vi "诊断标定4.vi"(8 "CAN端口":u16(ring), 9 "设备索引号":u16(ring), 10 "CAN卡类型":u32(ring)=4) -> ()   [LabVIEW 2013] (continued)
                n3070 = Build Array(i16 5 ("元素"), w4389, w4383, w4382, w4381, w4380, 0.0 ("元素")) -> (w4393:dbl[])
                n3071 = call "多帧发送机制(EV05).vi"("can卡类型"=w4397, "设备索引号"=w4396, "CAN端口"=w4395, "命令"=w4390, "板号"=u8 0, "命令序号"=w4379, "输入数据"=w4393) -> ()  [unwired: 1 in, 12 out]
              }
            }
            n3072 = local write "命令序号"(w4351) -> ()
            n3073 = local write "命令"(w4356) -> ()
            n3074 = local write "清BUFF"(FALSE ("清BUFF")) -> ()
            n3075 = local write "控制1"(TRUE ("控制1")) -> ()
            n3076 = global write "EV05全局变量1.vi" "流控帧 2"(FALSE ("流控帧 2")) -> ()
            n3077 = local write "写?"(FALSE ("写?")) -> ()
            n3078 = local write "消除"(TRUE ("消除")) -> ()
          }
          frame #2 {
            n3079 = flat-sequence {
              tunnel: [w4399] -> w4398
              tunnel: w4398 -> [w4406]
              frame #0 {
                n3080 = while {
                  tunnel: [w4400] -> w4399
                  i -> [w4404]
                  stop <- w4401 stop-if-true
                  n3081 = local read "继电器超时处理"() -> (w4400:bool)
                  n3082 = Greater Or Equal?(x=w4404, y=20) -> (x >= y?=w4402:bool)
                  n3083 = Wait Until Next ms Multiple(millisecond multiple=u32 100 ("毫秒倍数")) -> ()  [unwired: 1 out]
                  n3084 = Or(x=w4400, y=w4402) -> (x .or. y?=w4401:bool)
                }
              }
              frame #1 {
                n3085 = case shown="假" w4406 {
                  frame False {
                    n3086 = local read "充电继电器"() -> (w4407:bool)
                    n3087 = Not(x=w4407) -> (.not. x?=w4408:bool)
                    n3088 = local write "充电继电器"(w4408) -> ()
                    n3089 = One Button Dialog(message="继电器处理超时" ("消息"), button name ("OK")="是" ("按钮名称（“确定”）")) -> ()  [unwired: 1 out]
                  }
                  frame True {
                  }
                }
              }
            }
          }
        }
      }
      event "风机继电器": Value Change {
        n3090 = event-data() -> ("NewVal"=w4411:bool)  [unwired: 6 out]
        n3091 = stacked-sequence {
          tunnel: w4411 -> [_ w4423 _]
          frame #0 {
            w4414 = FALSE ("继电器超时处理")
            n3092 = local write "继电器超时处理"(w4414) -> ()
            n3093 = local write "正级继电器 6"(w4414) -> ()
            n3094 = local write "主从选择"(enum32{"主板", "从板"}."主板" ("主从选择")) -> ()
          }
          frame #1 {
            n3095 = case shown="真" w4423 {
              selector: w4423 -> [w4437 w4457]
              tunnel: [w4436 w4456] -> w4422
              tunnel: [w4425 w4445] -> w4417
              frame True {
                w4433 = 256.0 ("y")
                w4425 = u32 1 ("命令序号")
                w4436 = u8 192 ("命令")
                n3096 = local read "动作保持时间"() -> (w4434:dbl)
                n3097 = Quotient & Remainder(x=w4434, y=w4433) -> (x-y*floor(x/y)=w4426:dbl, floor(x/y)=w4430:dbl)
                n3098 = Quotient & Remainder(x=w4430, y=w4433) -> (x-y*floor(x/y)=w4427:dbl, floor(x/y)=w4431:dbl)
                n3099 = Quotient & Remainder(x=w4431, y=w4433) -> (x-y*floor(x/y)=w4428:dbl, floor(x/y)=w4432:dbl)
                n3100 = Boolean To (0,1)(Boolean=w4437) -> (0, 1=w4435:i16)
                n3101 = local read "设备索引号"() -> (w4442:u16)
                n3102 = local read "CAN卡类型"() -> (w4443:u32)
                n3103 = Quotient & Remainder(x=w4432, y=w4433) -> (x-y*floor(x/y)=w4429:dbl)  [unwired: 1 out]
                n3104 = local read "CAN端口"() -> (w4441:u16)
                n3105 = Build Array(i16 6 ("元素"), w4435, w4429, w4428, w4427, w4426, 0.0 ("元素")) -> (w4439:dbl[])
                n3106 = call "多帧发送机制(EV05).vi"("can卡类型"=w4443, "设备索引号"=w4442, "CAN端口"=w4441, "命令"=w4436, "板号"=u8 0, "命令序号"=w4425, "输入数据"=w4439) -> ()  [unwired: 1 in, 12 out]
              }
              frame False {
                w4453 = 256.0 ("y")
                w4445 = u32 1 ("命令序号")
                w4456 = u8 192 ("命令")
                n3107 = local read "动作保持时间"() -> (w4454:dbl)
                n3108 = Quotient & Remainder(x=w4454, y=w4453) -> (x-y*floor(x/y)=w4446:dbl, floor(x/y)=w4450:dbl)
                n3109 = Quotient & Remainder(x=w4450, y=w4453) -> (x-y*floor(x/y)=w4447:dbl, floor(x/y)=w4451:dbl)
                n3110 = Quotient & Remainder(x=w4451, y=w4453) -> (x-y*floor(x/y)=w4448:dbl, floor(x/y)=w4452:dbl)
                n3111 = Boolean To (0,1)(Boolean=w4457) -> (0, 1=w4455:i16)
                n3112 = local read "设备索引号"() -> (w4462:u16)
                n3113 = local read "CAN卡类型"() -> (w4463:u32)
                n3114 = Quotient & Remainder(x=w4452, y=w4453) -> (x-y*floor(x/y)=w4449:dbl)  [unwired: 1 out]
                n3115 = local read "CAN端口"() -> (w4461:u16)
                n3116 = Build Array(i16 6 ("元素"), w4455, w4449, w4448, w4447, w4446, 0.0 ("元素")) -> (w4459:dbl[])
                n3117 = call "多帧发送机制(EV05).vi"("can卡类型"=w4463, "设备索引号"=w4462, "CAN端口"=w4461, "命令"=w4456, "板号"=u8 0, "命令序号"=w4445, "输入数据"=w4459) -> ()  [unwired: 1 in, 12 out]
              }
            }
            n3118 = local write "命令序号"(w4417) -> ()
            n3119 = local write "命令"(w4422) -> ()
            n3120 = local write "清BUFF"(FALSE ("清BUFF")) -> ()
            n3121 = local write "控制1"(TRUE ("控制1")) -> ()
            n3122 = global write "EV05全局变量1.vi" "流控帧 2"(FALSE ("流控帧 2")) -> ()
            n3123 = local write "写?"(FALSE ("写?")) -> ()
            n3124 = local write "消除"(TRUE ("消除")) -> ()
          }
          frame #2 {
            n3125 = flat-sequence {
              tunnel: [w4465] -> w4464
              tunnel: w4464 -> [w4472]
              frame #0 {
                n3126 = while {
                  tunnel: [w4466] -> w4465
                  i -> [w4470]
                  stop <- w4467 stop-if-true
                  n3127 = local read "继电器超时处理"() -> (w4466:bool)
                  n3128 = Greater Or Equal?(x=w4470, y=20) -> (x >= y?=w4468:bool)
                  n3129 = Wait Until Next ms Multiple(millisecond multiple=u32 100 ("毫秒倍数")) -> ()  [unwired: 1 out]
                  n3130 = Or(x=w4466, y=w4468) -> (x .or. y?=w4467:bool)
                }
              }
              frame #1 {
                n3131 = case shown="假" w4472 {
                  frame False {
                    n3132 = local read "风机继电器"() -> (w4473:bool)
                    n3133 = Not(x=w4473) -> (.not. x?=w4474:bool)
                    n3134 = local write "风机继电器"(w4474) -> ()
                    n3135 = One Button Dialog(message="继电器处理超时" ("消息"), button name ("OK")="是" ("按钮名称（“确定”）")) -> ()  [unwired: 1 out]
                  }
                  frame True {
                  }
                }
              }
            }
          }
        }
      }
      event "加热继电器": Value Change {
        n3136 = event-data() -> ("NewVal"=w4477:bool)  [unwired: 6 out]
        n3137 = stacked-sequence {
          tunnel: w4477 -> [_ w4490 _]
          frame #0 {
            w4480 = FALSE ("继电器超时处理")
            n3138 = local write "正级继电器 7"(w4480) -> ()
            n3139 = local write "继电器超时处理"(w4480) -> ()
            n3140 = local write "主从选择"(enum32{"主板", "从板"}."从板" ("主从选择")) -> ()
          }
          frame #1 {
            n3141 = case shown="假" w4490 {
              selector: w4490 -> [w4505 w4525]
              tunnel: [w4504 w4524] -> w4489
              tunnel: [w4503 w4523] -> w4483
              tunnel: [w4492 w4512] -> w4484
              frame True {
                w4500 = 256.0 ("y")
                w4492 = u32 1 ("命令序号")
                w4504 = u8 192 ("命令")
                n3142 = local read "动作保持时间"() -> (w4501:dbl)
                n3143 = Quotient & Remainder(x=w4501, y=w4500) -> (x-y*floor(x/y)=w4493:dbl, floor(x/y)=w4497:dbl)
                n3144 = Quotient & Remainder(x=w4497, y=w4500) -> (x-y*floor(x/y)=w4494:dbl, floor(x/y)=w4498:dbl)
                n3145 = Quotient & Remainder(x=w4498, y=w4500) -> (x-y*floor(x/y)=w4495:dbl, floor(x/y)=w4499:dbl)
                n3146 = Quotient & Remainder(x=w4499, y=w4500) -> (x-y*floor(x/y)=w4496:dbl)  [unwired: 1 out]
                n3147 = Boolean To (0,1)(Boolean=w4505) -> (0, 1=w4502:i16)
                n3148 = local read "设备索引号"() -> (w4509:u16)
                n3149 = local read "CAN卡类型"() -> (w4510:u32)
                n3150 = local read "从板板号"() -> (w4503:u8)
                n3151 = local read "CAN端口"() -> (w4508:u16)
                n3152 = Build Array(i16 7 ("元素"), w4502, w4496, w4495, w4494, w4493, 0.0 ("元素")) -> (w4507:dbl[])
                n3153 = call "多帧发送机制(EV05).vi"("can卡类型"=w4510, "设备索引号"=w4509, "CAN端口"=w4508, "命令"=w4504, "板号"=w4503, "命令序号"=w4492, "输入数据"=w4507) -> ()  [unwired: 1 in, 12 out]
              }
              frame False {
                w4520 = 256.0 ("y")
                w4512 = u32 1 ("命令序号")
                w4524 = u8 192 ("命令")
                n3154 = local read "动作保持时间"() -> (w4521:dbl)
                n3155 = Quotient & Remainder(x=w4521, y=w4520) -> (x-y*floor(x/y)=w4513:dbl, floor(x/y)=w4517:dbl)
                n3156 = Quotient & Remainder(x=w4517, y=w4520) -> (x-y*floor(x/y)=w4514:dbl, floor(x/y)=w4518:dbl)
                n3157 = Quotient & Remainder(x=w4518, y=w4520) -> (x-y*floor(x/y)=w4515:dbl, floor(x/y)=w4519:dbl)
                n3158 = Quotient & Remainder(x=w4519, y=w4520) -> (x-y*floor(x/y)=w4516:dbl)  [unwired: 1 out]
                n3159 = Boolean To (0,1)(Boolean=w4525) -> (0, 1=w4522:i16)
                n3160 = local read "设备索引号"() -> (w4529:u16)
                n3161 = local read "CAN卡类型"() -> (w4530:u32)
                n3162 = local read "从板板号"() -> (w4523:u8)
                n3163 = local read "CAN端口"() -> (w4528:u16)
                n3164 = Build Array(i16 7 ("元素"), w4522, w4516, w4515, w4514, w4513, 0.0 ("元素")) -> (w4527:dbl[])
                n3165 = call "多帧发送机制(EV05).vi"("can卡类型"=w4530, "设备索引号"=w4529, "CAN端口"=w4528, "命令"=w4524, "板号"=w4523, "命令序号"=w4512, "输入数据"=w4527) -> ()  [unwired: 1 in, 12 out]
              }
            }
            n3166 = local write "从板板号"(w4483) -> ()
            n3167 = local write "命令序号"(w4484) -> ()
            n3168 = local write "命令"(w4489) -> ()
            n3169 = local write "清BUFF"(FALSE ("清BUFF")) -> ()
            n3170 = local write "写?"(FALSE ("写?")) -> ()
            n3171 = local write "控制1"(TRUE ("控制1")) -> ()
            n3172 = global write "EV05全局变量1.vi" "流控帧 2"(FALSE ("流控帧 2")) -> ()
            n3173 = local write "消除"(TRUE ("消除")) -> ()
          }
          frame #2 {
            n3174 = flat-sequence {
              tunnel: [w4532] -> w4531
              tunnel: w4531 -> [w4539]
              frame #0 {
                n3175 = while {
                  tunnel: [w4533] -> w4532
                  i -> [w4537]
                  stop <- w4534 stop-if-true
                  n3176 = local read "继电器超时处理"() -> (w4533:bool)
                  n3177 = Greater Or Equal?(x=w4537, y=20) -> (x >= y?=w4535:bool)
                  n3178 = Wait Until Next ms Multiple(millisecond multiple=u32 100 ("毫秒倍数")) -> ()  [unwired: 1 out]
                  n3179 = Or(x=w4533, y=w4535) -> (x .or. y?=w4534:bool)
                }
              }
              frame #1 {
                n3180 = case shown="假" w4539 {
                  frame False {
                    n3181 = local read "加热继电器"() -> (w4541:bool)
                    n3182 = Not(x=w4541) -> (.not. x?=w4540:bool)
                    n3183 = local write "加热继电器"(w4540) -> ()
                    n3184 = One Button Dialog(message="继电器处理超时" ("消息"), button name ("OK")="是" ("按钮名称（“确定”）")) -> ()  [unwired: 1 out]
                  }
                  frame True {
                  }
                }
              }
            }
          }
        }
      }
      event "风机继电器": Value Change {
        n3185 = event-data() -> ("NewVal"=w4544:bool)  [unwired: 6 out]
        n3186 = stacked-sequence {
          tunnel: w4544 -> [_ w4557 _]
          frame #0 {
            w4547 = FALSE ("继电器超时处理")
            n3187 = local write "继电器超时处理"(w4547) -> ()
            n3188 = local write "正级继电器 8"(w4547) -> ()
            n3189 = local write "主从选择"(enum32{"主板", "从板"}."从板" ("主从选择")) -> ()
          }
          frame #1 {
            n3190 = case shown="假" w4557 {
              selector: w4557 -> [w4572 w4592]
              tunnel: [w4571 w4591] -> w4556
              tunnel: [w4570 w4590] -> w4550
              tunnel: [w4559 w4579] -> w4551
              frame False {
                w4567 = 256.0 ("y")
                w4559 = u32 1 ("命令序号")
                w4571 = u8 192 ("命令")
                n3191 = local read "动作保持时间"() -> (w4568:dbl)
                n3192 = Quotient & Remainder(x=w4568, y=w4567) -> (x-y*floor(x/y)=w4560:dbl, floor(x/y)=w4564:dbl)
                n3193 = Quotient & Remainder(x=w4564, y=w4567) -> (x-y*floor(x/y)=w4561:dbl, floor(x/y)=w4565:dbl)
                n3194 = Quotient & Remainder(x=w4565, y=w4567) -> (x-y*floor(x/y)=w4562:dbl, floor(x/y)=w4566:dbl)
                n3195 = Quotient & Remainder(x=w4566, y=w4567) -> (x-y*floor(x/y)=w4563:dbl)  [unwired: 1 out]
                n3196 = local read "设备索引号"() -> (w4576:u16)
                n3197 = local read "CAN卡类型"() -> (w4577:u32)
                n3198 = local read "从板板号"() -> (w4570:u8)
                n3199 = Boolean To (0,1)(Boolean=w4572) -> (0, 1=w4569:i16)
                n3200 = local read "CAN端口"() -> (w4575:u16)
                n3201 = Build Array(i16 8 ("元素"), w4569, w4563, w4562, w4561, w4560, 0.0 ("元素")) -> (w4574:dbl[])
                n3202 = call "多帧发送机制(EV05).vi"("can卡类型"=w4577, "设备索引号"=w4576, "CAN端口"=w4575, "命令"=w4571, "板号"=w4570, "命令序号"=w4559, "输入数据"=w4574) -> ()  [unwired: 1 in, 12 out]
              }
              frame True {
                w4587 = 256.0 ("y")
                w4579 = u32 1 ("命令序号")
                w4591 = u8 192 ("命令")
                n3203 = local read "动作保持时间"() -> (w4588:dbl)
                n3204 = Quotient & Remainder(x=w4588, y=w4587) -> (x-y*floor(x/y)=w4580:dbl, floor(x/y)=w4584:dbl)
                n3205 = Quotient & Remainder(x=w4584, y=w4587) -> (x-y*floor(x/y)=w4581:dbl, floor(x/y)=w4585:dbl)
                n3206 = Quotient & Remainder(x=w4585, y=w4587) -> (x-y*floor(x/y)=w4582:dbl, floor(x/y)=w4586:dbl)
                n3207 = Quotient & Remainder(x=w4586, y=w4587) -> (x-y*floor(x/y)=w4583:dbl)  [unwired: 1 out]
                n3208 = local read "设备索引号"() -> (w4596:u16)
                n3209 = local read "CAN卡类型"() -> (w4597:u32)
                n3210 = local read "从板板号"() -> (w4590:u8)
                n3211 = Boolean To (0,1)(Boolean=w4592) -> (0, 1=w4589:i16)
                n3212 = local read "CAN端口"() -> (w4595:u16)
                n3213 = Build Array(i16 8 ("元素"), w4589, w4583, w4582, w4581, w4580, 0.0 ("元素")) -> (w4594:dbl[])
                n3214 = call "多帧发送机制(EV05).vi"("can卡类型"=w4597, "设备索引号"=w4596, "CAN端口"=w4595, "命令"=w4591, "板号"=w4590, "命令序号"=w4579, "输入数据"=w4594) -> ()  [unwired: 1 in, 12 out]
              }
            }
            n3215 = local write "从板板号"(w4550) -> ()
            n3216 = local write "清BUFF"(FALSE ("清BUFF")) -> ()
            n3217 = local write "命令序号"(w4551) -> ()
            n3218 = local write "命令"(w4556) -> ()
            n3219 = local write "控制1"(TRUE ("控制1")) -> ()
            n3220 = local write "写?"(FALSE ("写?")) -> ()
            n3221 = global write "EV05全局变量1.vi" "流控帧 2"(FALSE ("流控帧 2")) -> ()
            n3222 = local write "消除"(TRUE ("消除")) -> ()
          }
          frame #2 {
            n3223 = flat-sequence {
              tunnel: [w4599] -> w4598
              tunnel: w4598 -> [w4606]
              frame #0 {
                n3224 = while {
                  tunnel: [w4600] -> w4599
                  i -> [w4604]
                  stop <- w4601 stop-if-true
                  n3225 = local read "继电器超时处理"() -> (w4600:bool)
                  n3226 = Greater Or Equal?(x=w4604, y=20) -> (x >= y?=w4602:bool)
                  n3227 = Wait Until Next ms Multiple(millisecond multiple=u32 100 ("毫秒倍数")) -> ()  [unwired: 1 out]
                  n3228 = Or(x=w4600, y=w4602) -> (x .or. y?=w4601:bool)
                }
              }
              frame #1 {
                n3229 = case shown="假" w4606 {
                  frame False {
                    n3230 = local read "风机继电器"() -> (w4608:bool)
                    n3231 = Not(x=w4608) -> (.not. x?=w4607:bool)
                    n3232 = local write "风机继电器"(w4607) -> ()
                    n3233 = One Button Dialog(message="继电器处理超时" ("消息"), button name ("OK")="是" ("按钮名称（“确定”）")) -> ()  [unwired: 1 out]
                  }
                  frame True {
                  }
                }
              }
            }
          }
        }
      }
      event "DO1": Value Change {
        n3234 = event-data() -> ("NewVal"=w4611:bool)  [unwired: 6 out]
        n3235 = stacked-sequence {
          tunnel: w4611 -> [_ w4623 _]
          frame #0 {
            w4614 = FALSE ("清BUFF")
            n3236 = local write "继电器超时处理"(FALSE ("继电器超时处理")) -> ()
            n3237 = local write "清BUFF"(w4614) -> ()
            n3238 = local write "正级继电器 9"(w4614) -> ()
            n3239 = local write "主从选择"(enum32{"主板", "从板"}."主板" ("主从选择")) -> ()
          }
          frame #1 {
            n3240 = case shown="假" w4623 {
              selector: w4623 -> [w4638 w4658]
              tunnel: [w4637 w4657] -> w4622
              tunnel: [w4625 w4645] -> w4617
              frame False {
                w4633 = 256.0 ("y")
                w4625 = u32 2 ("命令序号")
                w4637 = u8 192 ("命令")
                n3241 = local read "动作保持时间"() -> (w4634:dbl)
                n3242 = Quotient & Remainder(x=w4634, y=w4633) -> (x-y*floor(x/y)=w4626:dbl, floor(x/y)=w4630:dbl)
                n3243 = Quotient & Remainder(x=w4630, y=w4633) -> (x-y*floor(x/y)=w4627:dbl, floor(x/y)=w4631:dbl)
                n3244 = local read "设备索引号"() -> (w4642:u16)
                n3245 = Quotient & Remainder(x=w4631, y=w4633) -> (x-y*floor(x/y)=w4628:dbl, floor(x/y)=w4632:dbl)
                n3246 = local read "CAN卡类型"() -> (w4643:u32)
                n3247 = local read "CAN端口"() -> (w4641:u16)
                n3248 = Boolean To (0,1)(Boolean=w4638) -> (0, 1=w4635:i16)
                n3249 = Quotient & Remainder(x=w4632, y=w4633) -> (x-y*floor(x/y)=w4629:dbl)  [unwired: 1 out]
                n3250 = Build Array(i16 1 ("元素"), w4635, w4629, w4628, w4627, w4626, 0.0 ("元素")) -> (w4639:dbl[])
                n3251 = call "多帧发送机制(EV05).vi"("can卡类型"=w4643, "设备索引号"=w4642, "CAN端口"=w4641, "命令"=w4637, "板号"=u8 0, "命令序号"=w4625, "输入数据"=w4639) -> ()  [unwired: 1 in, 12 out]
              }
              frame True {
                w4653 = 256.0 ("y")
                w4645 = u32 2 ("命令序号")
                w4657 = u8 192 ("命令")
                n3252 = local read "动作保持时间"() -> (w4654:dbl)
                n3253 = Quotient & Remainder(x=w4654, y=w4653) -> (x-y*floor(x/y)=w4646:dbl, floor(x/y)=w4650:dbl)
                n3254 = Quotient & Remainder(x=w4650, y=w4653) -> (x-y*floor(x/y)=w4647:dbl, floor(x/y)=w4651:dbl)
                n3255 = local read "设备索引号"() -> (w4662:u16)
                n3256 = Quotient & Remainder(x=w4651, y=w4653) -> (x-y*floor(x/y)=w4648:dbl, floor(x/y)=w4652:dbl)
                n3257 = local read "CAN卡类型"() -> (w4663:u32)
                n3258 = local read "CAN端口"() -> (w4661:u16)
                n3259 = Boolean To (0,1)(Boolean=w4658) -> (0, 1=w4655:i16)
                n3260 = Quotient & Remainder(x=w4652, y=w4653) -> (x-y*floor(x/y)=w4649:dbl)  [unwired: 1 out]
                n3261 = Build Array(i16 1 ("元素"), w4655, w4649, w4648, w4647, w4646, 0.0 ("元素")) -> (w4659:dbl[])
                n3262 = call "多帧发送机制(EV05).vi"("can卡类型"=w4663, "设备索引号"=w4662, "CAN端口"=w4661, "命令"=w4657, "板号"=u8 0, "命令序号"=w4645, "输入数据"=w4659) -> ()  [unwired: 1 in, 12 out]
              }
            }
            n3263 = local write "命令序号"(w4617) -> ()
            n3264 = local write "命令"(w4622) -> ()
            n3265 = local write "控制1"(TRUE ("控制1")) -> ()
            n3266 = local write "写?"(FALSE ("写?")) -> ()
            n3267 = global write "EV05全局变量1.vi" "流控帧 2"(FALSE ("流控帧 2")) -> ()
            n3268 = local write "消除"(TRUE ("消除")) -> ()
          }
          frame #2 {
            n3269 = flat-sequence {
              tunnel: [w4665] -> w4664
              tunnel: w4664 -> [w4672]
              frame #0 {
                n3270 = while {
                  tunnel: [w4666] -> w4665
                  i -> [w4670]
                  stop <- w4667 stop-if-true
                  n3271 = local read "继电器超时处理"() -> (w4666:bool)
                  n3272 = Greater Or Equal?(x=w4670, y=20) -> (x >= y?=w4668:bool)
                  n3273 = Wait Until Next ms Multiple(millisecond multiple=u32 100 ("毫秒倍数")) -> ()  [unwired: 1 out]
                  n3274 = Or(x=w4666, y=w4668) -> (x .or. y?=w4667:bool)
                }
              }
              frame #1 {
                n3275 = case shown="假" w4672 {
                  frame False {
                    n3276 = local read "DO1"() -> (w4674:bool)
                    n3277 = Not(x=w4674) -> (.not. x?=w4673:bool)
                    n3278 = local write "DO1"(w4673) -> ()
                    n3279 = One Button Dialog(message="DO控制处理超时" ("消息"), button name ("OK")="是" ("按钮名称（“确定”）")) -> ()  [unwired: 1 out]
                  }
                  frame True {
                  }
                }
              }
            }
          }
        }
      }
      event "DO2": Value Change {
        n3280 = event-data() -> ("NewVal"=w4677:bool)  [unwired: 6 out]
        n3281 = stacked-sequence {
          tunnel: w4677 -> [_ w4689 _]
          frame #0 {
            w4680 = FALSE ("清BUFF")
            n3282 = local write "继电器超时处理"(FALSE ("继电器超时处理")) -> ()
            n3283 = local write "主从选择"(enum32{"主板", "从板"}."主板" ("主从选择")) -> ()
            n3284 = local write "清BUFF"(w4680) -> ()
            n3285 = local write "正级继电器 10"(w4680) -> ()
          }
          frame #1 {
            n3286 = case shown="假" w4689 {
              selector: w4689 -> [w4704 w4724]
              tunnel: [w4703 w4723] -> w4688
              tunnel: [w4691 w4711] -> w4683
              frame False {
                w4699 = 256.0 ("y")
                w4691 = u32 2 ("命令序号")
                w4703 = u8 192 ("命令")
                n3287 = local read "动作保持时间"() -> (w4700:dbl)
                n3288 = Quotient & Remainder(x=w4700, y=w4699) -> (x-y*floor(x/y)=w4692:dbl, floor(x/y)=w4696:dbl)
                n3289 = Quotient & Remainder(x=w4696, y=w4699) -> (x-y*floor(x/y)=w4693:dbl, floor(x/y)=w4697:dbl)
                n3290 = local read "设备索引号"() -> (w4708:u16)
                n3291 = Quotient & Remainder(x=w4697, y=w4699) -> (x-y*floor(x/y)=w4694:dbl, floor(x/y)=w4698:dbl)
                n3292 = local read "CAN卡类型"() -> (w4709:u32)
                n3293 = local read "CAN端口"() -> (w4707:u16)
                n3294 = Boolean To (0,1)(Boolean=w4704) -> (0, 1=w4701:i16)
                n3295 = Quotient & Remainder(x=w4698, y=w4699) -> (x-y*floor(x/y)=w4695:dbl)  [unwired: 1 out]
                n3296 = Build Array(i16 2 ("元素"), w4701, w4695, w4694, w4693, w4692, 0.0 ("元素")) -> (w4705:dbl[])
                n3297 = call "多帧发送机制(EV05).vi"("can卡类型"=w4709, "设备索引号"=w4708, "CAN端口"=w4707, "命令"=w4703, "板号"=u8 0, "命令序号"=w4691, "输入数据"=w4705) -> ()  [unwired: 1 in, 12 out]
              }
              frame True {
                w4719 = 256.0 ("y")
                w4711 = u32 2 ("命令序号")
                w4723 = u8 192 ("命令")
                n3298 = local read "动作保持时间"() -> (w4720:dbl)
                n3299 = Quotient & Remainder(x=w4720, y=w4719) -> (x-y*floor(x/y)=w4712:dbl, floor(x/y)=w4716:dbl)
                n3300 = Quotient & Remainder(x=w4716, y=w4719) -> (x-y*floor(x/y)=w4713:dbl, floor(x/y)=w4717:dbl)
                n3301 = local read "设备索引号"() -> (w4728:u16)
                n3302 = Quotient & Remainder(x=w4717, y=w4719) -> (x-y*floor(x/y)=w4714:dbl, floor(x/y)=w4718:dbl)
                n3303 = local read "CAN卡类型"() -> (w4729:u32)
                n3304 = local read "CAN端口"() -> (w4727:u16)
                n3305 = Boolean To (0,1)(Boolean=w4724) -> (0, 1=w4721:i16)
                n3306 = Quotient & Remainder(x=w4718, y=w4719) -> (x-y*floor(x/y)=w4715:dbl)  [unwired: 1 out]
                n3307 = Build Array(i16 2 ("元素"), w4721, w4715, w4714, w4713, w4712, 0.0 ("元素")) -> (w4725:dbl[])
                n3308 = call "多帧发送机制(EV05).vi"("can卡类型"=w4729, "设备索引号"=w4728, "CAN端口"=w4727, "命令"=w4723, "板号"=u8 0, "命令序号"=w4711, "输入数据"=w4725) -> ()  [unwired: 1 in, 12 out]
              }
            }
            n3309 = local write "命令序号"(w4683) -> ()
            n3310 = local write "命令"(w4688) -> ()
            n3311 = local write "控制1"(TRUE ("控制1")) -> ()
            n3312 = local write "写?"(FALSE ("写?")) -> ()
            n3313 = global write "EV05全局变量1.vi" "流控帧 2"(FALSE ("流控帧 2")) -> ()
            n3314 = local write "消除"(TRUE ("消除")) -> ()
          }
          frame #2 {
            n3315 = flat-sequence {
              tunnel: [w4731] -> w4730
              tunnel: w4730 -> [w4738]
              frame #0 {
                n3316 = while {
                  tunnel: [w4732] -> w4731
                  i -> [w4736]
                  stop <- w4733 stop-if-true
                  n3317 = local read "继电器超时处理"() -> (w4732:bool)
                  n3318 = Greater Or Equal?(x=w4736, y=20) -> (x >= y?=w4734:bool)
                  n3319 = Wait Until Next ms Multiple(millisecond multiple=u32 100 ("毫秒倍数")) -> ()  [unwired: 1 out]
                  n3320 = Or(x=w4732, y=w4734) -> (x .or. y?=w4733:bool)
                }
              }
              frame #1 {
                n3321 = case shown="假" w4738 {
                  frame False {
                    n3322 = local read "DO2"() -> (w4740:bool)
                    n3323 = Not(x=w4740) -> (.not. x?=w4739:bool)
                    n3324 = local write "DO2"(w4739) -> ()
                    n3325 = One Button Dialog(message="DO控制处理超时" ("消息"), button name ("OK")="是" ("按钮名称（“确定”）")) -> ()  [unwired: 1 out]
                  }
                  frame True {
                  }
                }
              }
            }
          }
        }
      }
      event "DO1 2": Value Change {
        n3326 = event-data() -> ("NewVal"=w4743:bool)  [unwired: 6 out]
        n3327 = stacked-sequence {
          tunnel: w4743 -> [_ w4756 _]
          frame #0 {
            w4746 = FALSE ("继电器超时处理")
            n3328 = local write "继电器超时处理"(w4746) -> ()
            n3329 = local write "正级继电器 11"(w4746) -> ()
            n3330 = local write "主从选择"(enum32{"主板", "从板"}."从板" ("主从选择")) -> ()
          }
          frame #1 {
            n3331 = case shown="假" w4756 {
              selector: w4756 -> [w4771 w4791]
              tunnel: [w4770 w4790] -> w4755
              tunnel: [w4769 w4789] -> w4749
              tunnel: [w4758 w4778] -> w4750
              frame True {
                w4766 = 256.0 ("y")
                w4758 = u32 2 ("命令序号")
                w4770 = u8 192 ("命令")
                n3332 = local read "动作保持时间"() -> (w4767:dbl)
                n3333 = Quotient & Remainder(x=w4767, y=w4766) -> (x-y*floor(x/y)=w4759:dbl, floor(x/y)=w4763:dbl)
                n3334 = Quotient & Remainder(x=w4763, y=w4766) -> (x-y*floor(x/y)=w4760:dbl, floor(x/y)=w4764:dbl)
                n3335 = Quotient & Remainder(x=w4764, y=w4766) -> (x-y*floor(x/y)=w4761:dbl, floor(x/y)=w4765:dbl)
                n3336 = Quotient & Remainder(x=w4765, y=w4766) -> (x-y*floor(x/y)=w4762:dbl)  [unwired: 1 out]
                n3337 = Boolean To (0,1)(Boolean=w4771) -> (0, 1=w4768:i16)
                n3338 = local read "设备索引号"() -> (w4775:u16)
                n3339 = local read "CAN卡类型"() -> (w4776:u32)
                n3340 = local read "从板板号"() -> (w4769:u8)
                n3341 = local read "CAN端口"() -> (w4774:u16)
                n3342 = Build Array(i16 3 ("元素"), w4768, w4762, w4761, w4760, w4759, 0.0 ("元素")) -> (w4773:dbl[])
                n3343 = call "多帧发送机制(EV05).vi"("can卡类型"=w4776, "设备索引号"=w4775, "CAN端口"=w4774, "命令"=w4770, "板号"=w4769, "命令序号"=w4758, "输入数据"=w4773) -> ()  [unwired: 1 in, 12 out]
              }
              frame False {
                w4786 = 256.0 ("y")
                w4778 = u32 2 ("命令序号")
                w4790 = u8 192 ("命令")
                n3344 = local read "动作保持时间"() -> (w4787:dbl)
                n3345 = Quotient & Remainder(x=w4787, y=w4786) -> (x-y*floor(x/y)=w4779:dbl, floor(x/y)=w4783:dbl)
                n3346 = Quotient & Remainder(x=w4783, y=w4786) -> (x-y*floor(x/y)=w4780:dbl, floor(x/y)=w4784:dbl)
                n3347 = Quotient & Remainder(x=w4784, y=w4786) -> (x-y*floor(x/y)=w4781:dbl, floor(x/y)=w4785:dbl)
                n3348 = Quotient & Remainder(x=w4785, y=w4786) -> (x-y*floor(x/y)=w4782:dbl)  [unwired: 1 out]
                n3349 = Boolean To (0,1)(Boolean=w4791) -> (0, 1=w4788:i16)
                n3350 = local read "设备索引号"() -> (w4795:u16)
                n3351 = local read "CAN卡类型"() -> (w4796:u32)
                n3352 = local read "从板板号"() -> (w4789:u8)
                n3353 = local read "CAN端口"() -> (w4794:u16)
                n3354 = Build Array(i16 1 ("元素"), w4788, w4782, w4781, w4780, w4779, 0.0 ("元素")) -> (w4793:dbl[])
                n3355 = call "多帧发送机制(EV05).vi"("can卡类型"=w4796, "设备索引号"=w4795, "CAN端口"=w4794, "命令"=w4790, "板号"=w4789, "命令序号"=w4778, "输入数据"=w4793) -> ()  [unwired: 1 in, 12 out]
              }
            }
            n3356 = local write "从板板号"(w4749) -> ()
            n3357 = local write "命令序号"(w4750) -> ()
            n3358 = local write "命令"(w4755) -> ()
            n3359 = local write "清BUFF"(FALSE ("清BUFF")) -> ()
            n3360 = local write "写?"(FALSE ("写?")) -> ()
            n3361 = local write "控制1"(TRUE ("控制1")) -> ()
            n3362 = global write "EV05全局变量1.vi" "流控帧 2"(FALSE ("流控帧 2")) -> ()
            n3363 = local write "消除"(TRUE ("消除")) -> ()
          }
          frame #2 {
            n3364 = flat-sequence {
              tunnel: [w4798] -> w4797
              tunnel: w4797 -> [w4805]
              frame #0 {
                n3365 = while {
                  tunnel: [w4799] -> w4798
                  i -> [w4803]
                  stop <- w4800 stop-if-true
                  n3366 = local read "继电器超时处理"() -> (w4799:bool)
                  n3367 = Greater Or Equal?(x=w4803, y=20) -> (x >= y?=w4801:bool)
                  n3368 = Wait Until Next ms Multiple(millisecond multiple=u32 100 ("毫秒倍数")) -> ()  [unwired: 1 out]
                  n3369 = Or(x=w4799, y=w4801) -> (x .or. y?=w4800:bool)
                }
              }
              frame #1 {
                n3370 = case shown="假" w4805 {
                  frame False {
                    n3371 = local read "DO1 2"() -> (w4807:bool)
                    n3372 = Not(x=w4807) -> (.not. x?=w4806:bool)
                    n3373 = local write "DO1 2"(w4806) -> ()
                    n3374 = One Button Dialog(message="DO控制处理超时" ("消息"), button name ("OK")="是" ("按钮名称（“确定”）")) -> ()  [unwired: 1 out]
                  }
                  frame True {
                  }
                }
              }
            }
          }
        }
      }
      event "读取转换为写入": Value Change {
        n3375 = event-data() -> ("NewVal"=w4810:bool)  [unwired: 6 out]
        n3376 = case shown="真" w4810 {
          tunnel: w4814 -> [w4816 w4821]
          tunnel: [w4816 w4820] -> w4813
          tunnel: w4812 -> [w4815 w4819]
          tunnel: [w4815 w4818] -> w4811
          frame False {
          }
          frame True {
            n3377 = Enqueue Element(queue=w4821, element="读取转换为写入", error in (no error)=w4819) -> (queue out=w4820:refnum<queue>, error out=w4818:errorcluster)  [unwired: 2 out]
          }
        }
      }
      event "读取故障详细状态": Value Change {
        n3378 = event-data() -> ("NewVal"=w4826:bool)  [unwired: 5 out]
        n3379 = case shown="真" w4826 {
          tunnel: w4825 -> [w4828 w4840]
          tunnel: w4824 -> [w4827 w4839]
          tunnel: [w4828 w4838] -> w4823
          tunnel: [w4827 w4837] -> w4822
          frame False {
          }
          frame True {
            n3380 = disable-structure shown="启用" {
              disable-tunnel: [w4849 TRUE ("发送成功")] -> w4836
              frame Disabled {
                n3381 = local read "主从选择"() -> (w4841:enum32{"主板", "从板"})
                n3382 = case shown="\"主板\", 默认" w4841 {
                  tunnel: [0.0 ("FUNC") w4851] -> w4846
                  frame "主板", Default {
                  }
                  frame "从板" {
                    n3383 = local read "从板板号"() -> (w4851:u8)
                  }
                }
                n3384 = local read "设备索引号"() -> (w4843:u16)
                n3385 = local read "CAN卡类型"() -> (w4844:u32)
                n3386 = local read "CAN端口"() -> (w4842:u16)
                n3387 = call "标定授权发送.vi"("CAN卡类型"=w4844, "解锁类型"=enum16{"读取", "写", "下载"}."写", "设备索引号"=w4843, "CAN端口"=w4842, "是否连接"=TRUE, "板选择"=0, "FUNC"=w4846) -> ("发送成功"=w4849:bool)  [unwired: 8 out]
              }
              frame Enabled {
              }
            }
            n3388 = case shown="真" w4836 {
              tunnel: w4840 -> [w4854 w4859]
              tunnel: w4839 -> [w4853 w4858]
              tunnel: [w4854 w4856] -> w4838
              tunnel: [w4853 w4855] -> w4837
              frame False {
              }
              frame True {
                n3389 = Enqueue Element(queue=w4859, element="读取故障状态" ("元素"), error in (no error)=w4858) -> (queue out=w4856:refnum<queue>, error out=w4855:errorcluster)  [unwired: 2 out]
              }
            }
            n3390 = local write "电池故障"(string[][] []) -> ()
            n3391 = local write "写?"(TRUE ("写?")) -> ()
            n3392 = local write "控制1"(TRUE ("控制1")) -> ()
            n3393 = local write "消除"(TRUE ("消除")) -> ()
            n3394 = global write "EV05全局变量1.vi" "流控帧 2"(FALSE ("流控帧 2")) -> ()
            n3395 = local write "清BUFF"(FALSE ("清BUFF")) -> ()
            n3396 = call <vilib>:"Set Busy.vi"("disable click? (T)"=FALSE) -> ()  [unwired: 3 in, 8 out]
          }
        }
      }
      event "项目软本读取": Value Change {
        n3397 = event-data() -> ("NewVal"=w4864:bool)  [unwired: 5 out]
        n3398 = case shown="真" w4864 {
          tunnel: w4863 -> [w4866 w4873]
          tunnel: w4862 -> [w4865 w4872]
          tunnel: [w4866 w4871] -> w4861
          tunnel: [w4865 w4870] -> w4860
          frame False {
          }
          frame True {
            n3399 = global read "EV05全局变量1.vi" "授权功能"() -> (w4868:bool)
            n3400 = case shown="假" w4868 {
              tunnel: [TRUE ("发送成功") w4891] -> w4869
              frame False {
              }
              frame True {
                n3401 = local read "设备索引号"() -> (w4886:u16)
                n3402 = local read "CAN卡类型"() -> (w4887:u32)
                n3403 = local read "CAN端口"() -> (w4885:u16)
                n3404 = call "标定授权发送.vi"("CAN卡类型"=w4887, "解锁类型"=enum16{"读取", "写", "下载"}."读取", "设备索引号"=w4886, "CAN端口"=w4885, "是否连接"=TRUE, "板选择"=0, "FUNC"=u32 0) -> ("发送成功"=w4891:bool)  [unwired: 8 out]
              }
            }
            n3405 = stacked-sequence {
              tunnel: [w4875] -> w4867
              frame #0 {
                w4875 = FALSE ("disable click? (T)")
                w4878 = FALSE ("写?")
                n3406 = local write "写?"(w4878) -> ()
                n3407 = global write "EV05全局变量1.vi" "写入超时"(w4878) -> ()
                n3408 = local write "项目软件版本号"(" " ("项目软件版本号")) -> ()
                n3409 = local write "主从选择"(enum32{"主板", "从板"}."主板" ("主从选择")) -> ()
                n3410 = call <vilib>:"Set Busy.vi"("disable click? (T)"=w4875) -> ()  [unwired: 3 in, 8 out]
                n3411 = property on="保存版本信息" class="Bool (严格)"("Visible"=TRUE ("可见")) -> ()  [unwired: 2 in, 2 out]
                n3412 = local write "清BUFF"(FALSE ("清BUFF")) -> ()
                n3413 = global write "EV05全局变量1.vi" "流控帧 2"(FALSE ("流控帧 2")) -> ()
                n3414 = local write "控制1"(TRUE ("控制1")) -> ()
                n3415 = local write "消除"(TRUE ("消除")) -> ()
              }
            }
            n3416 = case shown="真" w4869 {
              tunnel: w4873 -> [w4893 w4898]
              tunnel: w4872 -> [w4892 w4897]
              tunnel: [w4893 w4895] -> w4871
              tunnel: [w4892 w4894] -> w4870
              tunnel: w4867 -> [_ _]
              frame False {
              }
              frame True {
                n3417 = Enqueue Element(queue=w4898, element="项目软件版本读取" ("元素"), error in (no error)=w4897) -> (queue out=w4895:refnum<queue>, error out=w4894:errorcluster)  [unwired: 2 out]
              }
            }
          }
        }
      }
      event "读硬件版本号": Value Change {
        n3418 = event-data() -> ("NewVal"=w4903:bool)  [unwired: 5 out]
        n3419 = case shown="真" w4903 {
          tunnel: w4902 -> [w4905 w4912]
          tunnel: w4901 -> [w4904 w4911]
          tunnel: [w4905 w4910] -> w4900
          tunnel: [w4904 w4909] -> w4899
          frame False {
          }
          frame True {
            n3420 = global read "EV05全局变量1.vi" "授权功能"() -> (w4907:bool)
            n3421 = case shown="假" w4907 {
              tunnel: [TRUE ("发送成功") w4930] -> w4908
              frame False {
              }
              frame True {
                n3422 = local read "设备索引号"() -> (w4925:u16)
                n3423 = local read "CAN卡类型"() -> (w4926:u32)
                n3424 = local read "CAN端口"() -> (w4924:u16)
                n3425 = call "标定授权发送.vi"("CAN卡类型"=w4926, "解锁类型"=enum16{"读取", "写", "下载"}."读取", "设备索引号"=w4925, "CAN端口"=w4924, "是否连接"=TRUE, "板选择"=0, "FUNC"=u32 0) -> ("发送成功"=w4930:bool)  [unwired: 8 out]
              }
            }
            n3426 = stacked-sequence {
              tunnel: [w4914] -> w4906
              frame #0 {
                w4914 = TRUE ("控制1")
                w4918 = FALSE ("写?")
                n3427 = local write "写?"(w4918) -> ()
                n3428 = global write "EV05全局变量1.vi" "写入超时"(w4918) -> ()
                n3429 = call <vilib>:"Set Busy.vi"("disable click? (T)"=FALSE) -> ()  [unwired: 3 in, 8 out]
                n3430 = local write "硬件版本号"("" ("硬件版本号")) -> ()
                n3431 = property on="保存版本信息" class="Bool (严格)"("Visible"=TRUE ("可见")) -> ()  [unwired: 2 in, 2 out]
                n3432 = local write "主从选择"(enum32{"主板", "从板"}."主板" ("主从选择")) -> ()
                n3433 = global write "EV05全局变量1.vi" "流控帧 2"(FALSE ("流控帧 2")) -> ()
                n3434 = local write "控制1"(w4914) -> ()
                n3435 = local write "清BUFF"(FALSE ("清BUFF")) -> ()
                n3436 = local write "消除"(TRUE ("消除")) -> ()
              }
            }
            n3437 = case shown="真" w4908 {
              tunnel: w4912 -> [w4932 w4937]
              tunnel: w4911 -> [w4931 w4936]
              tunnel: [w4932 w4934] -> w4910
              tunnel: [w4931 w4933] -> w4909
              tunnel: w4906 -> [_ _]
              frame False {
              }
              frame True {
                n3438 = Enqueue Element(queue=w4937, element="硬件版本读取" ("元素"), error in (no error)=w4936) -> (queue out=w4934:refnum<queue>, error out=w4933:errorcluster)  [unwired: 2 out]
              }
            }
          }
        }
      }
      event "平台软件版本读取": Value Change {
        n3439 = event-data() -> ("NewVal"=w4942:bool)  [unwired: 5 out]
        n3440 = case shown="真" w4942 {
          tunnel: w4941 -> [w4944 w4951]
          tunnel: w4940 -> [w4943 w4950]
          tunnel: [w4944 w4949] -> w4939
          tunnel: [w4943 w4948] -> w4938
          frame False {
          }
          frame True {
            n3441 = global read "EV05全局变量1.vi" "授权功能"() -> (w4946:bool)
            n3442 = case shown="假" w4946 {
              tunnel: [TRUE ("发送成功") w4969] -> w4947
              frame False {
              }
              frame True {
                n3443 = local read "设备索引号"() -> (w4964:u16)
                n3444 = local read "CAN卡类型"() -> (w4965:u32)
                n3445 = local read "CAN端口"() -> (w4963:u16)
                n3446 = call "标定授权发送.vi"("CAN卡类型"=w4965, "解锁类型"=enum16{"读取", "写", "下载"}."读取", "设备索引号"=w4964, "CAN端口"=w4963, "是否连接"=TRUE, "板选择"=0, "FUNC"=u32 0) -> ("发送成功"=w4969:bool)  [unwired: 8 out]
              }
            }
            n3447 = stacked-sequence {
              tunnel: [w4953] -> w4945
              frame #0 {
                w4953 = TRUE ("控制1")
                w4957 = FALSE ("写?")
                n3448 = call <vilib>:"Set Busy.vi"("disable click? (T)"=FALSE) -> ()  [unwired: 3 in, 8 out]
                n3449 = local write "写?"(w4957) -> ()
                n3450 = global write "EV05全局变量1.vi" "写入超时"(w4957) -> ()
                n3451 = local write "平台软件版本号"(" " ("平台软件版本号")) -> ()
                n3452 = local write "控制1"(w4953) -> ()
                n3453 = local write "消除"(TRUE ("消除")) -> ()
                n3454 = property on="保存版本信息" class="Bool (严格)"("Visible"=TRUE ("可见")) -> ()  [unwired: 2 in, 2 out]
                n3455 = global write "EV05全局变量1.vi" "流控帧 2"(FALSE ("流控帧 2")) -> ()
                n3456 = local write "主从选择"(enum32{"主板", "从板"}."主板" ("主从选择")) -> ()
                n3457 = local write "清BUFF"(FALSE ("清BUFF")) -> ()
              }
            }
            n3458 = case shown="真" w4947 {
              tunnel: w4951 -> [w4971 w4976]
              tunnel: w4950 -> [w4970 w4975]
              tunnel: [w4971 w4973] -> w4949
              tunnel: [w4970 w4972] -> w4948
              tunnel: w4945 -> [_ _]
              frame False {
              }
              frame True {
                n3459 = Enqueue Element(queue=w4976, element="平台软件版本读取" ("元素"), error in (no error)=w4975) -> (queue out=w4973:refnum<queue>, error out=w4972:errorcluster)  [unwired: 2 out]
              }
            }
          }
        }
      }
      event "模块版本读取": Value Change {
        n3460 = event-data() -> ("NewVal"=w4981:bool)  [unwired: 5 out]
        n3461 = case shown="真" w4981 {
          tunnel: w4980 -> [w4983 w4990]
          tunnel: w4979 -> [w4982 w4989]
          tunnel: [w4983 w4988] -> w4978
          tunnel: [w4982 w4987] -> w4977
          frame False {
          }
          frame True {
            n3462 = global read "EV05全局变量1.vi" "授权功能"() -> (w4985:bool)
            n3463 = case shown="假" w4985 {
              tunnel: [TRUE ("发送成功") w5007] -> w4986
              frame False {
              }
              frame True {
                n3464 = local read "设备索引号"() -> (w5002:u16)
                n3465 = local read "CAN卡类型"() -> (w5003:u32)
                n3466 = local read "CAN端口"() -> (w5001:u16)
                n3467 = call "标定授权发送.vi"("CAN卡类型"=w5003, "解锁类型"=enum16{"读取", "写", "下载"}."读取", "设备索引号"=w5002, "CAN端口"=w5001, "是否连接"=TRUE, "板选择"=0, "FUNC"=u32 0) -> ("发送成功"=w5007:bool)  [unwired: 8 out]
              }
            }
            n3468 = stacked-sequence {
              tunnel: [w4992] -> w4984
              frame #0 {
                w4992 = TRUE ("控制1")
                w4995 = FALSE ("写?")
                n3469 = call <vilib>:"Set Busy.vi"("disable click? (T)"=FALSE) -> ()  [unwired: 3 in, 8 out]
                n3470 = local write "写?"(w4995) -> ()
                n3471 = global write "EV05全局变量1.vi" "写入超时"(w4995) -> ()
                n3472 = local write "主从选择"(enum32{"主板", "从板"}."主板" ("主从选择")) -> ()
                n3473 = property on="保存版本信息" class="Bool (严格)"("Visible"=TRUE ("可见")) -> ()  [unwired: 2 in, 2 out]
                n3474 = local write "清BUFF"(FALSE ("清BUFF")) -> ()
                n3475 = global write "EV05全局变量1.vi" "流控帧 2"(FALSE ("流控帧 2")) -> ()
                n3476 = local write "控制1"(w4992) -> ()
                n3477 = local write "消除"(TRUE ("消除")) -> ()
              }
            }
            n3478 = case shown="真" w4986 {
              tunnel: w4990 -> [w5009 w5014]
              tunnel: w4989 -> [w5008 w5013]
              tunnel: [w5009 w5011] -> w4988
              tunnel: [w5008 w5010] -> w4987
              tunnel: w4984 -> [_ _]
              frame False {
              }
              frame True {
                n3479 = Enqueue Element(queue=w5014, element="模块软件版本读取" ("元素"), error in (no error)=w5013) -> (queue out=w5011:refnum<queue>, error out=w5010:errorcluster)  [unwired: 2 out]
              }
            }
          }
        }
      }
      event "保存版本信息": Value Change {
        n3480 = event-data() -> ("NewVal"=w5015:bool)  [unwired: 6 out]
        n3481 = case shown="真" w5015 {
          frame False {
          }
          frame True {
            n3482 = stacked-sequence {
              seq-local: [w5019 _] -> [_ w5021]
              seq-local: [w5018 _] -> [_ w5020]
              frame #0 {
                n3483 = call "请输入从板个数"() -> ("从板个数"=w5019:dbl, "确定"=w5018:bool)  [unwired: 17 in, 1 out]
              }
              frame #1 {
                n3484 = case shown="真" w5020 {
                  tunnel: w5021 -> [_ w5024]
                  frame False {
                  }
                  frame True {
                    n3485 = call <vilib>:"Application Directory.vi"() -> ("Application Directory"=w5036:path)
                    n3486 = Build Path(base path=w5036, name or relative path="SaveData" ("名称或相对路径")) -> (appended path=w5034:path)
                    n3487 = local read "模块版本名称"() -> (w5029:string[][])
                    n3488 = local read "项目软件版本"() -> (w5026:string[])
                    n3489 = local read "模块版本值"() -> (w5028:string[][])
                    n3490 = local read "平台软件版本"() -> (w5025:string[])
                    n3491 = local read "模块个数"() -> (w5022:u8[])
                    n3492 = local read "硬件版本"() -> (w5027:string[])
                    n3493 = call "文件对话框3"("start path"=w5034, "prompt"="选择要保存数据的位置", "default name"="BMS版本信息.txt") -> ("selected path"=w5030:path, "cancelled"=w5031:bool)  [unwired: 9 in, 2 out]
                    n3494 = Increment(x=w5024) -> (x+1=w5023:dbl)
                    n3495 = for {
                      N: w5023 -> [_]
                      tunnel: w5031 -> [w5052]
                      tunnel: w5030 -> [w5051]
                      tunnel: w5029 -> [w5041] mode=indexing
                      tunnel: w5028 -> [w5039] mode=indexing
                      tunnel: w5027 -> [w5046] mode=indexing
                      tunnel: w5026 -> [w5045] mode=indexing
                      tunnel: w5025 -> [w5044] mode=indexing
                      tunnel: w5022 -> [w5037] mode=indexing
                      i -> [w5043]
                      w5049 = ""
                      w5056 = 0 ("索引")
                      n3496 = case shown="0, 默认" w5043 {
                        selector: w5043 -> [_ w5070]
                        tunnel: ["主板版本信息" w5071] -> w5061
                        tunnel: [FALSE TRUE] -> w5047
                        frame 0, Default {
                        }
                        frame 1.. {
                          n3497 = Number To Decimal String(number=w5070) -> (decimal integer string=w5069:string)  [unwired: 1 in]
                          n3498 = Concatenate Strings("从板", w5069, "版本信息") -> (w5071:string)
                        }
                      }
                      n3499 = Increment(x=w5037) -> (x+1=w5038:u8)
                      n3500 = Array Subset(array=w5041, length=w5038) -> (w5042:string[])  [unwired: 1 in]
                      n3501 = Array Subset(array=w5039, length=w5038) -> (w5040:string[])  [unwired: 1 in]
                      n3502 = Build Array(w5049, w5044, w5045, w5046, w5049) -> (w5055:string[])
                      n3503 = Build Array(w5061, "平台软件版本号", "项目软件版本号", "硬件版本号", "模块版本号") -> (w5057:string[])
                      n3504 = Insert Into Array(array=w5042, index=w5056, new element=w5057) -> (w5054:string[])
                      n3505 = Insert Into Array(array=w5040, index=w5056, new element=w5055) -> (w5053:string[])
                      n3506 = Build Array(w5054, w5053) -> (w5050:string[][])
                      n3507 = case shown="假" w5052 {
                        tunnel: w5051 -> [w5065 _]
                        tunnel: w5050 -> [w5064 _]
                        tunnel: w5047 -> [w5062 _]
                        frame False {
                          n3508 = call-poly <vilib>:"Write To Spreadsheet File.vi"("transpose? (no:F)"=TRUE, "append to file? (new file:F)"=w5062, "2D data"=w5064, "file path (dialog if empty)"=w5065) -> ()  [unwired: 4 in, 1 out]
                        }
                        frame True {
                        }
                      }
                    }
                  }
                }
              }
            }
          }
        }
      }
      event "单个写入": Value Change {
        n3509 = event-data() -> ("NewVal"=w5078:bool)  [unwired: 5 out]
        n3510 = case shown="真" w5078 {
          tunnel: w5077 -> [w5080 w5092]
          tunnel: w5076 -> [w5079 w5091]
          tunnel: [w5080 w5090] -> w5075
          tunnel: [w5079 w5089] -> w5074
          frame False {
          }
          frame True {
            n3511 = disable-structure shown="启用" {
              disable-tunnel: [w5101 TRUE ("发送成功")] -> w5088
              frame Disabled {
                n3512 = local read "主从选择"() -> (w5093:enum32{"主板", "从板"})
                n3513 = case shown="\"主板\", 默认" w5093 {
                  tunnel: [0.0 ("FUNC") w5103] -> w5098
                  frame "主板", Default {
                  }
                  frame "从板" {
                    n3514 = local read "从板板号"() -> (w5103:u8)
                  }
                }
                n3515 = local read "设备索引号"() -> (w5095:u16)
                n3516 = local read "CAN卡类型"() -> (w5096:u32)
                n3517 = local read "CAN端口"() -> (w5094:u16)
                n3518 = call "标定授权发送.vi"("CAN卡类型"=w5096, "解锁类型"=enum16{"读取", "写", "下载"}."写", "设备索引号"=w5095, "CAN端口"=w5094, "是否连接"=TRUE, "板选择"=0, "FUNC"=w5098) -> ("发送成功"=w5101:bool)  [unwired: 8 out]
              }
              frame Enabled {
              }
            }
            n3519 = case shown="真" w5088 {
              tunnel: w5092 -> [w5106 w5111]
              tunnel: w5091 -> [w5105 w5110]
              tunnel: [w5106 w5108] -> w5090
              tunnel: [w5105 w5107] -> w5089
              frame False {
              }
              frame True {
                n3520 = Enqueue Element(queue=w5111, element="单个写入" ("元素"), error in (no error)=w5110) -> (queue out=w5108:refnum<queue>, error out=w5107:errorcluster)  [unwired: 2 out]
              }
            }
            n3521 = global write "EV05全局变量1.vi" "流控帧 2"(FALSE ("流控帧 2")) -> ()
            n3522 = local write "写?"(TRUE ("写?")) -> ()
            n3523 = local write "控制1"(TRUE ("控制1")) -> ()
            n3524 = local write "消除"(TRUE ("消除")) -> ()
            n3525 = local write "清BUFF"(FALSE ("清BUFF")) -> ()
            n3526 = global write "EV05全局变量1.vi" "输出数组"(u8[] [] ("输出数组")) -> ()
            n3527 = call <vilib>:"Set Busy.vi"("disable click? (T)"=FALSE) -> ()  [unwired: 3 in, 8 out]
          }
        }
      }
      event "全部写入": Value Change {
        n3528 = event-data() -> ("NewVal"=w5116:bool)  [unwired: 5 out]
        n3529 = case shown="真" w5116 {
          tunnel: w5115 -> [w5118 w5131]
          tunnel: w5114 -> [w5117 w5130]
          tunnel: [w5118 w5129] -> w5113
          tunnel: [w5117 w5128] -> w5112
          frame False {
          }
          frame True {
            n3530 = global read "EV05全局变量1.vi" "授权功能"() -> (w5123:bool)
            n3531 = case shown="假" w5123 {
              tunnel: [TRUE ("发送成功") w5141] -> w5127
              frame False {
              }
              frame True {
                n3532 = local read "主从选择"() -> (w5133:enum32{"主板", "从板"})
                n3533 = case shown="\"从板\"" w5133 {
                  tunnel: [0.0 ("FUNC") w5143] -> w5134
                  frame "主板", Default {
                  }
                  frame "从板" {
                    n3534 = local read "从板板号"() -> (w5143:u8)
                  }
                }
                n3535 = local read "设备索引号"() -> (w5136:u16)
                n3536 = local read "CAN卡类型"() -> (w5137:u32)
                n3537 = local read "CAN端口"() -> (w5135:u16)
                n3538 = call "标定授权发送.vi"("CAN卡类型"=w5137, "解锁类型"=enum16{"读取", "写", "下载"}."写", "设备索引号"=w5136, "CAN端口"=w5135, "是否连接"=TRUE, "板选择"=0, "FUNC"=w5134) -> ("发送成功"=w5141:bool)  [unwired: 8 out]
              }
            }
            n3539 = case shown="真" w5127 {
              tunnel: w5131 -> [w5145 w5150]
              tunnel: w5130 -> [w5144 w5149]
              tunnel: [w5145 w5147] -> w5129
              tunnel: [w5144 w5146] -> w5128
              frame False {
              }
              frame True {
                n3540 = Enqueue Element(queue=w5150, element="全部写入" ("元素"), error in (no error)=w5149) -> (queue out=w5147:refnum<queue>, error out=w5146:errorcluster)  [unwired: 2 out]
              }
            }
            n3541 = local write "写?"(TRUE ("写?")) -> ()
            n3542 = global write "EV05全局变量1.vi" "输出数组"(u8[] [] ("输出数组")) -> ()
            n3543 = local write "清BUFF"(FALSE ("清BUFF")) -> ()
            n3544 = local write "控制1"(TRUE ("控制1")) -> ()
            n3545 = global write "EV05全局变量1.vi" "流控帧 2"(FALSE ("流控帧 2")) -> ()
            n3546 = local write "消除"(TRUE ("消除")) -> ()
            n3547 = call <vilib>:"Set Busy.vi"("disable click? (T)"=FALSE) -> ()  [unwired: 3 in, 8 out]
          }
        }
      }
      event "单个读取": Value Change {
        n3548 = event-data() -> ("NewVal"=w5155:bool)  [unwired: 5 out]
        n3549 = case shown="真" w5155 {
          tunnel: w5154 -> [w5157 w5170]
          tunnel: w5153 -> [w5156 w5169]
          tunnel: [w5157 w5168] -> w5152
          tunnel: [w5156 w5167] -> w5151
          frame False {
          }
          frame True {
            n3550 = global read "EV05全局变量1.vi" "授权功能"() -> (w5163:bool)
            n3551 = case shown="假" w5163 {
              tunnel: [TRUE ("发送成功") w5179] -> w5166
              frame False {
              }
              frame True {
